vi "Start.vi"(8 "error in (no error)":errorcluster, 11 "EventDaemon in":refnum<class "ErrorHandler.lvclass">) -> (0 "error out":errorcluster, 3 "EventDaemon out":refnum<class "ErrorHandler.lvclass">)   [LabVIEW 2024, in "ErrorHandler.lvclass"]
doc: "Runs daemon asynchronously"
uses:
  ErrorHandler.lvclass
  ErrorHandler.lvclass/ErrorHandler.ctl
  private/daemon.vi
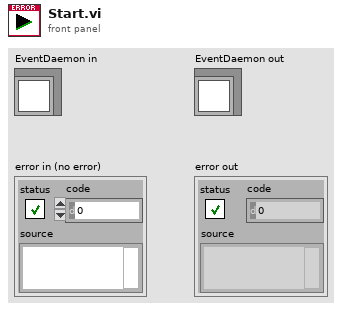
[diagram p1: front panel]
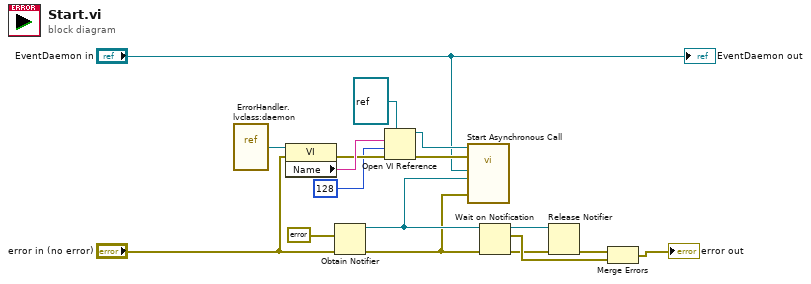
[diagram p0: block diagram]
diagram:
  n1 = vi-ref "ErrorHandler.lvclass:daemon.vi"() -> (w17:refnum<vi>)
  n2 = property class="VI"(reference=w17, error in="error in (no error)") -> (error out=w15:errorcluster, "Name"=w16:string)  [unwired: 1 out]
  n3 = Obtain Notifier(notification data type=errorcluster {"status"=FALSE, "code"=0, "source"=""} ("error in (no error)"), error in (no error)="error in (no error)") -> (notifier out=w7:refnum<notifier>, error out=w6:errorcluster)  [unwired: 2 in, 1 out]
  n4 = Open VI Reference(type specifier VI Refnum (for type only)=refnum<vi> refnum, vi path=w16, options=128, error in (no error)=w15) -> (vi reference=w12:refnum<vi>, error out=w11:errorcluster)  [unwired: 2 in]
  n5 = call-by-ref "Start Asynchronous Call"(reference=w12, error in=w11, 8:"error in (no error)"=w6, "callback notifier"=w7, "EventDaemon.lvclass"="EventDaemon in") -> ()  [unwired: 8 in, 3 out]
  n6 = Wait on Notification(notifier=w7, error in (no error)=w6) -> (notifier out=w1:refnum<notifier>, notification=w5:errorcluster, error out=w2:errorcluster)  [unwired: 2 in, 1 out]
  n7 = Release Notifier(notifier=w1, error in (no error)=w2) -> (error out=w3:errorcluster)  [unwired: 1 in, 2 out]
  n8 = Merge Errors(w3, w5) -> (→"error out":errorcluster)
  "EventDaemon out" <- "EventDaemon in"
